vi "Stem Page.vi"() -> ()   [LabVIEW 2020, in "3D Stem.lvclass"]
uses:
  <vilib>/Math Plots/3D Math Plots/3D Stem/3D Stem/3D Stem.lvclass
  <vilib>/Math Plots/3D Math Plots/3D Stem/3D Stem/Typedef/3D Stem Property Array.ctl
  <vilib>/Math Plots/3D Math Plots/3D Stem/3D Stem/Typedef/3D Stem Property.ctl
  <vilib>/Math Plots/3D Math Plots/3D Plot/3D Plot/Typedef/Sprite Type.ctl
  <vilib>/Math Plots/3D Math Plots/3D Plot/3D Plot/Typedef/Color Ramp Cluster.ctl
  <vilib>/Math Plots/3D Math Plots/3D Plot/3D Plot/Typedef/Line Type.ctl
  <vilib>/Math Plots/3D Math Plots/3D Plot/3D Plot/Typedef/Dialog State.ctl
  <vilib>/Math Plots/3D Math Plots/3D Plot/3D Plot/Typedef/Temp Scene State.ctl
  <vilib>/Math Plots/3D Math Plots/3D Plot/3D Plot/Typedef/Temp Scene Property Action.ctl
  <vilib>/Math Plots/3D Math Plots/3D Plot/3D Plot/3D Plot.lvclass
panel:
  in  "Point Size":sgl caption="Point size" min=0.001 step=1
  in  "Point Style":u16(ring) caption="Point style"
  in  "Line Width":sgl=0.001 caption="Line width" min=0.001 step=1
  in  "Antialiasing":bool
  in  "Line Style":u16(ring) caption="Line style"
  in  "Line Color":u32(colorbox) caption="Line color"
  out "Stem Property Out":T1
  in  "Stem Property In":T1
  out "Color Ramp":dbl[][](graph)
  in  "Color Map Style":u16(ring) caption="Color map style" items=["None ", "Shaded", "Color spectrum", "Grey scale", "Custom"]
  in  "YZ Plane Projection":bool caption="YZ plane projection"
  in  "XZ Plane Projection":bool caption="XZ plane projection"
  in  "XY Plane Projection":bool caption="XY  plane projection"
  in  "Coordinate System":u16(ring) caption="Coordinate system" items=["Cartesian", "Cylindrical", "Spherical"]
  in  "Plot Opacity":sgl(slide) caption="Plot opacity(%)" min=0 max=100 scale=0.0..100.0
  in  "Plot List":i32(listbox)
  in  "Ramp Edit":bool caption="Ramp edit"
  in  "Move Down":bool
  in  "Move Up":bool
  in  "Delete":bool
  in  "New":bool
  in  "Event Registration":refnum<event-registration>
  # "Stem"
  # "General"
  # "Projection"
  # "Color Ramp"
  # "Stem Line"
  # "Stem Point"
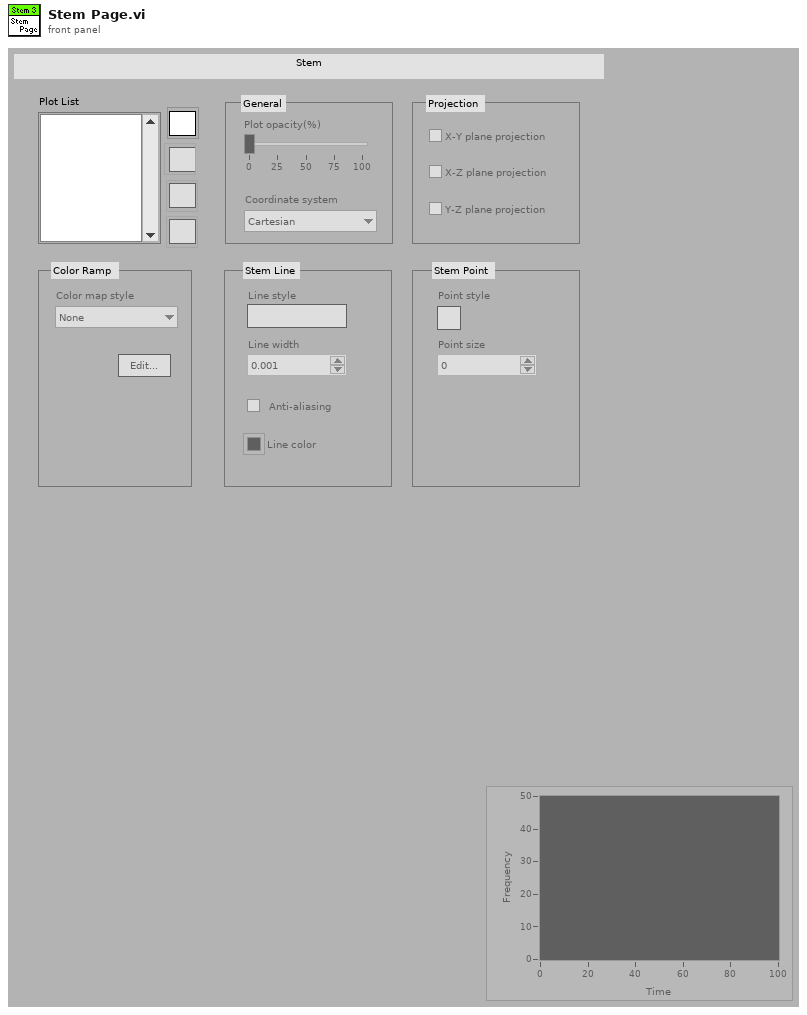
[diagram p1: front panel]
types:
  T1 = typedef "3D Stem.lvclass/3D Stem Property Array.ctl" = T2[]
  T2 = typedef "3D Stem.lvclass/3D Stem Property.ctl" = cluster{"General Property":cluster{"Plot Name":string, "Coordinate System":enum16{"Cartesian", "Cylindrical", "Spherical"}, "Opacity":sgl}, "Projection Property":cluster{"Draw XY":bool, "Draw YZ":bool, "Draw XZ":bool}, "Plot Property":cluster{"Sprite Type":T3, "Point Size":sgl, "Color Ramp Cluster":T4, "Line Style":T5, "Line Width":sgl, "Line Color":u32, "Antialiasing":bool}}
  T3 = typedef "3D Plot.lvclass/Sprite Type.ctl" = enum16{"None", "Empty Square", "Solid Square", "Empty Diamond", "Solid Diamond", "Empty Circle", "Solid Circle", "Asterisk", "Bold X", "Wireframe Sphere", "Solid Sphere", "Wireframe Cube", "Solid Cube"}
  T4 = typedef "3D Plot.lvclass/Color Ramp Cluster.ctl" = cluster{"Color Ramp Style":enum16{"None", "Shaded", "Color spectrum", "Grey scale", "Custom"}, "Color Ramp Array":u32[], "Color Ramp Index":i32[], "Interpolate?":bool, "Logarithm?":bool}
  T5 = typedef "3D Plot.lvclass/Line Type.ctl" = enum16{"None", "Solid", "Dash", "Dot", "Dash Dot"}
  T6 = typedef "3D Plot.lvclass/Dialog State.ctl" = enum16{"Initialize", "Read Porperty", "Write Property", "Idle", "Exit"}
  T7 = typedef "3D Plot.lvclass/Temp Scene State.ctl" = enum16{"Create", "Update Scene", "Get Plot Representation", "Destory"}
  T8 = typedef "3D Plot.lvclass/Temp Scene Property Action.ctl" = enum16{"Graph Property", "Light Property", "Axis Property", "Value Pair Property", "Format Property", "Cursor Property", "Plot Specific Property"}
  T9 = typedef "3D Plot.lvclass/Multiplot Representation.ctl" = cluster{"Plot Represention Array":T10[], "Max Range":T11}
  T10 = typedef "3D Plot.lvclass/Plot Representation.ctl" = cluster{"Plot ID":i32, "Plot Range":T11, "Mesh Data":T12, "Dimension":cluster{"X Dimension":i32, "Y Dimension":i32}, "Ramp Range":T11}
  T11 = typedef "3D Plot.lvclass/Range Clusters.ctl" = cluster{"X Range":cluster{"Max X":sgl, "Min X":sgl}, "Y Range":cluster{"Max Y":sgl, "Min Y":sgl}, "Z Range":cluster{"Max Z":sgl, "Min Z":sgl}}
  T12 = typedef "3D Plot.lvclass/Mesh Data.ctl" = cluster{"Index Array":u32[], "Vertex Array":cluster{"X":sgl, "Y":sgl, "Z":sgl}[], "Normal Array":cluster{"X":sgl, "Y":sgl, "Z":sgl}[], "Color Index Array":i32[]}
  T13 = enum16{"None", "Shaded", "Color spectrum", "Grey scale", "Custom"}
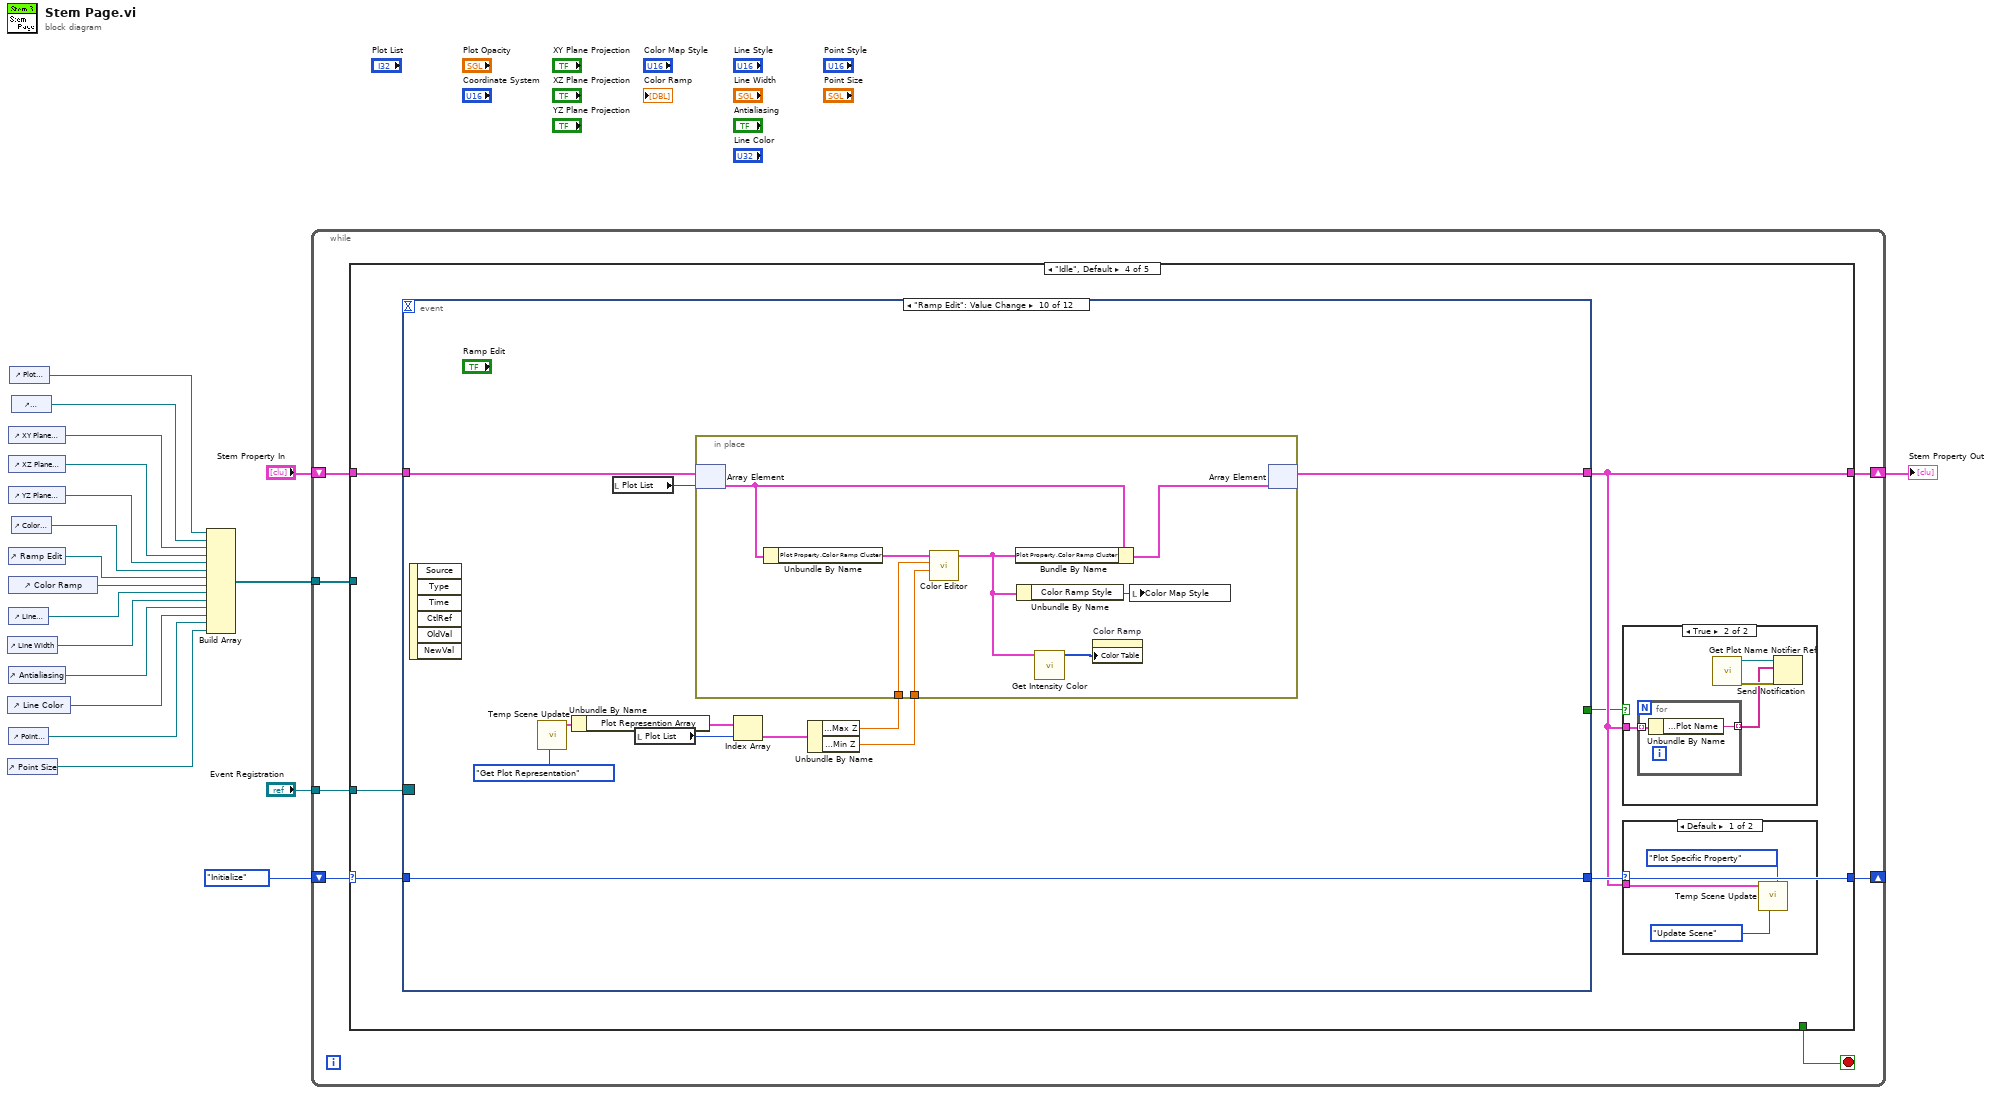
[diagram p0: block diagram]
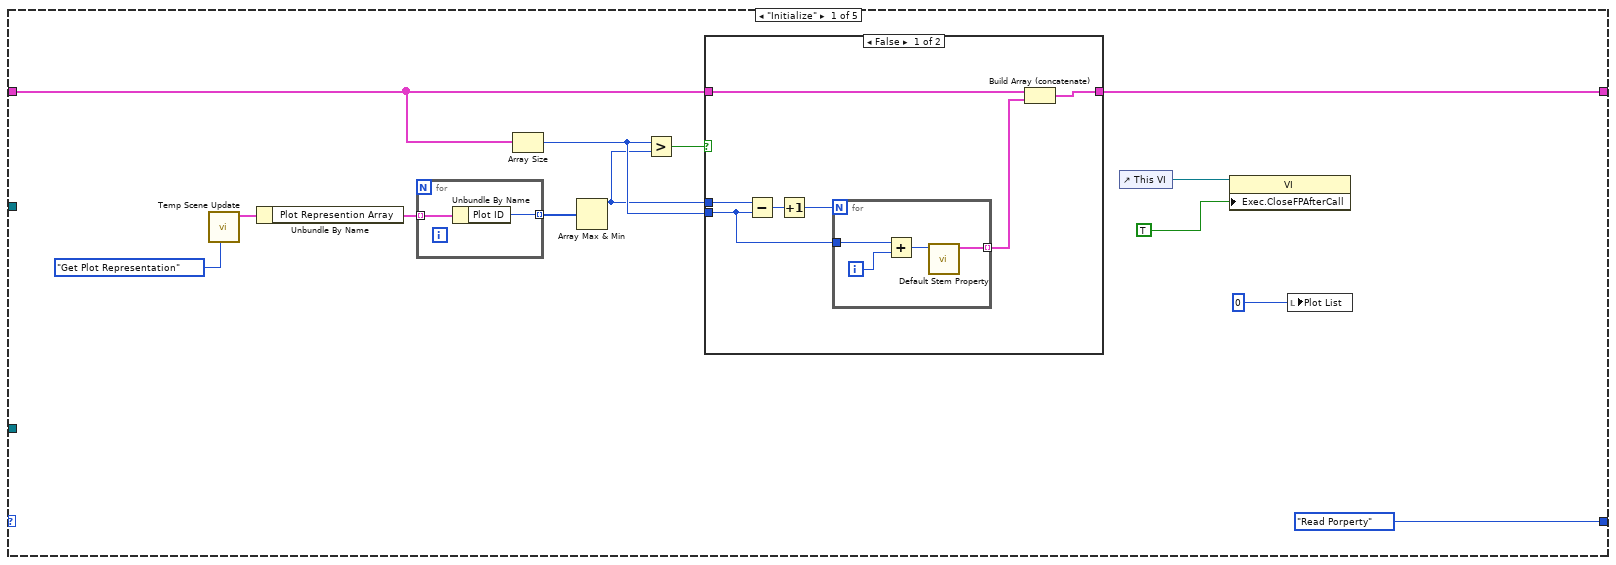
[diagram p2: hidden frame]
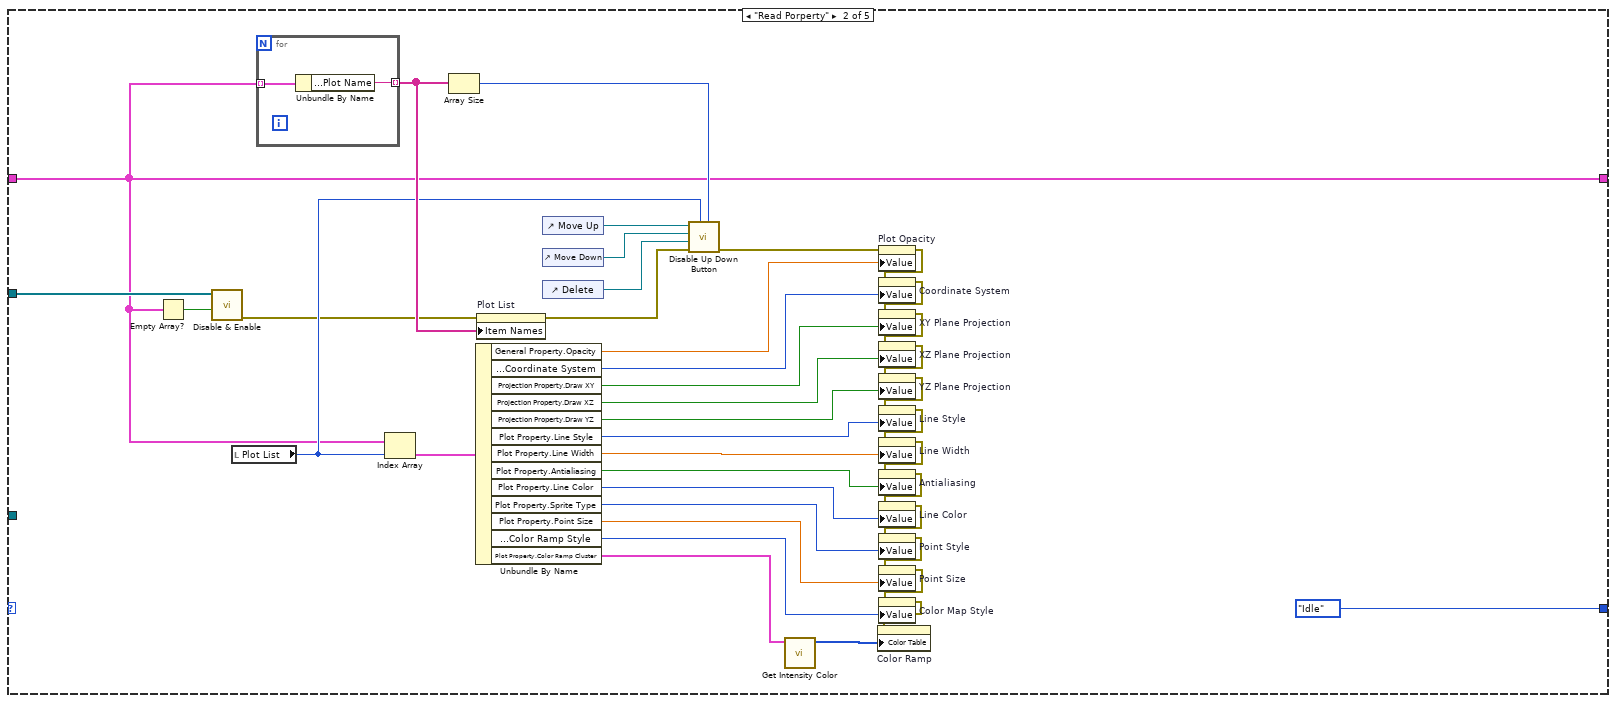
[diagram p4: hidden frame]
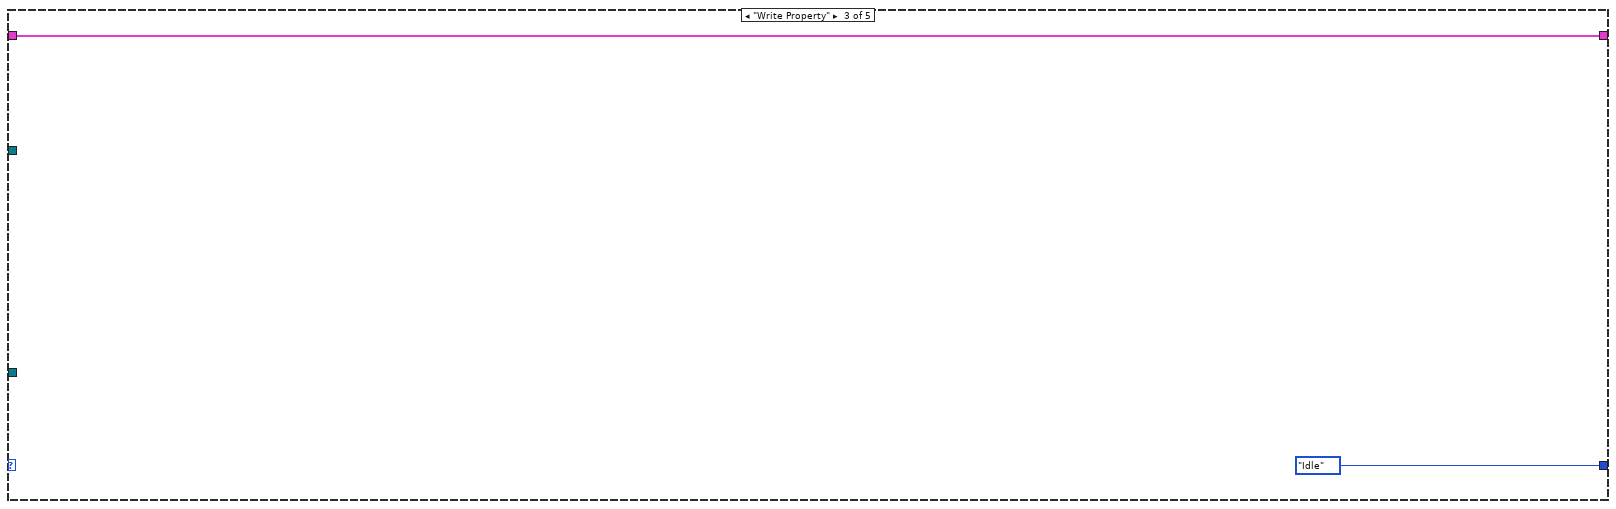
[diagram p5: hidden frame]
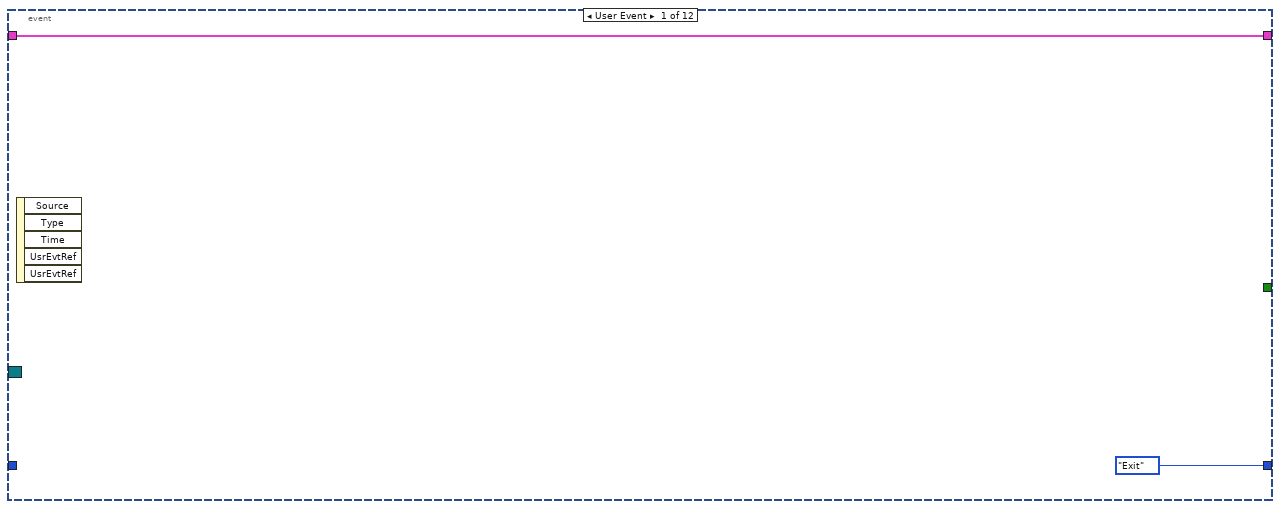
[diagram p8: hidden frame]
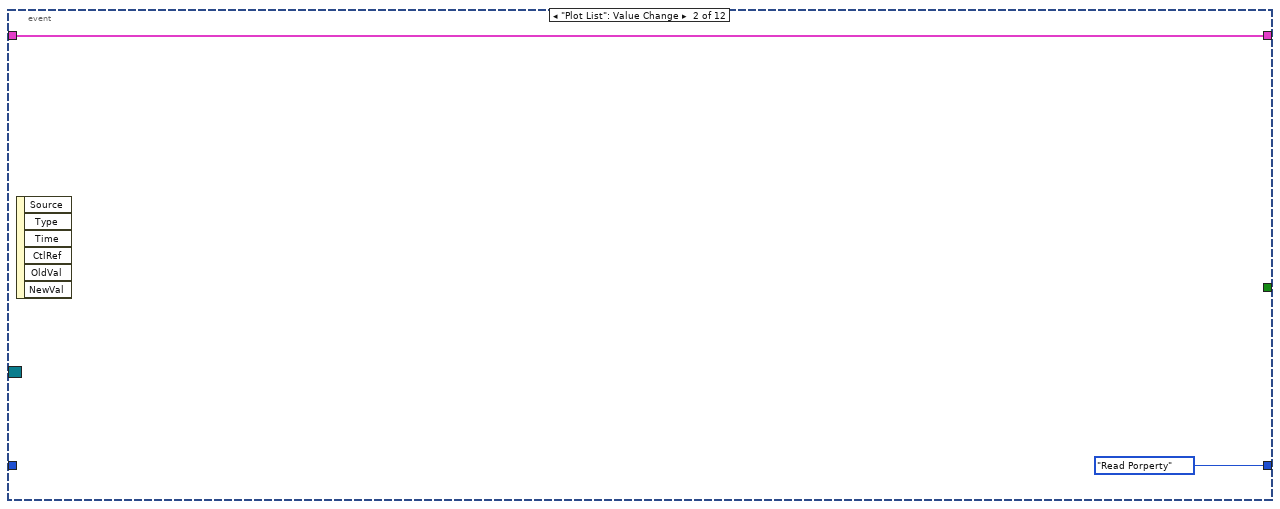
[diagram p9: hidden frame]
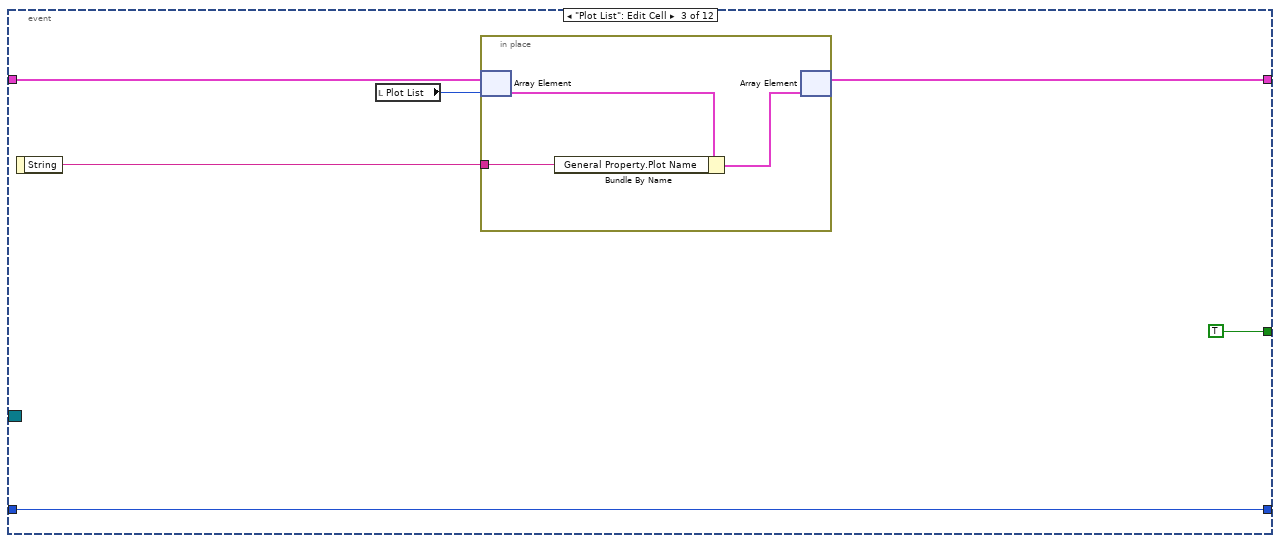
[diagram p10: hidden frame]
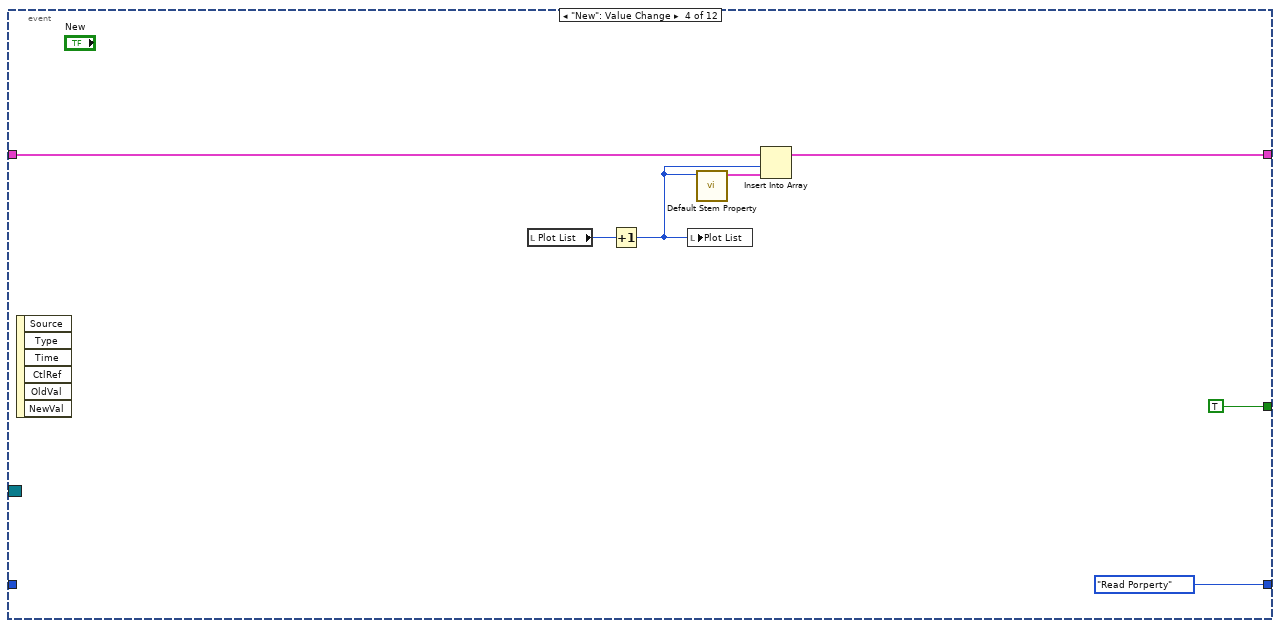
[diagram p11: hidden frame]
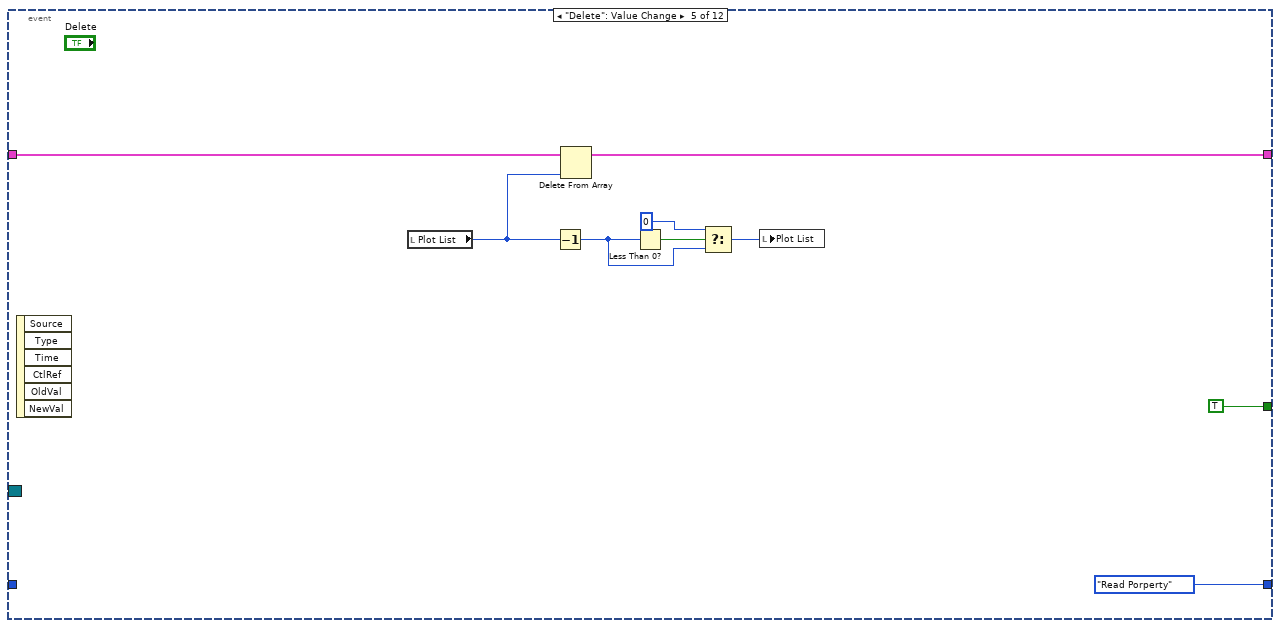
[diagram p12: hidden frame]
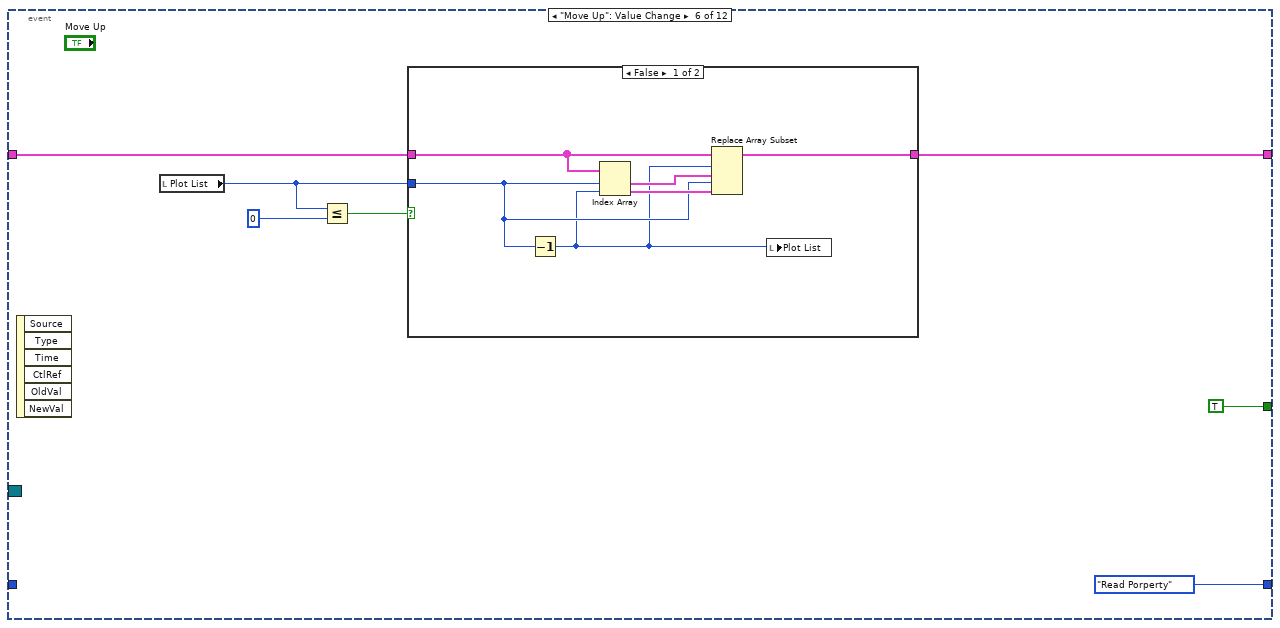
[diagram p13: hidden frame]
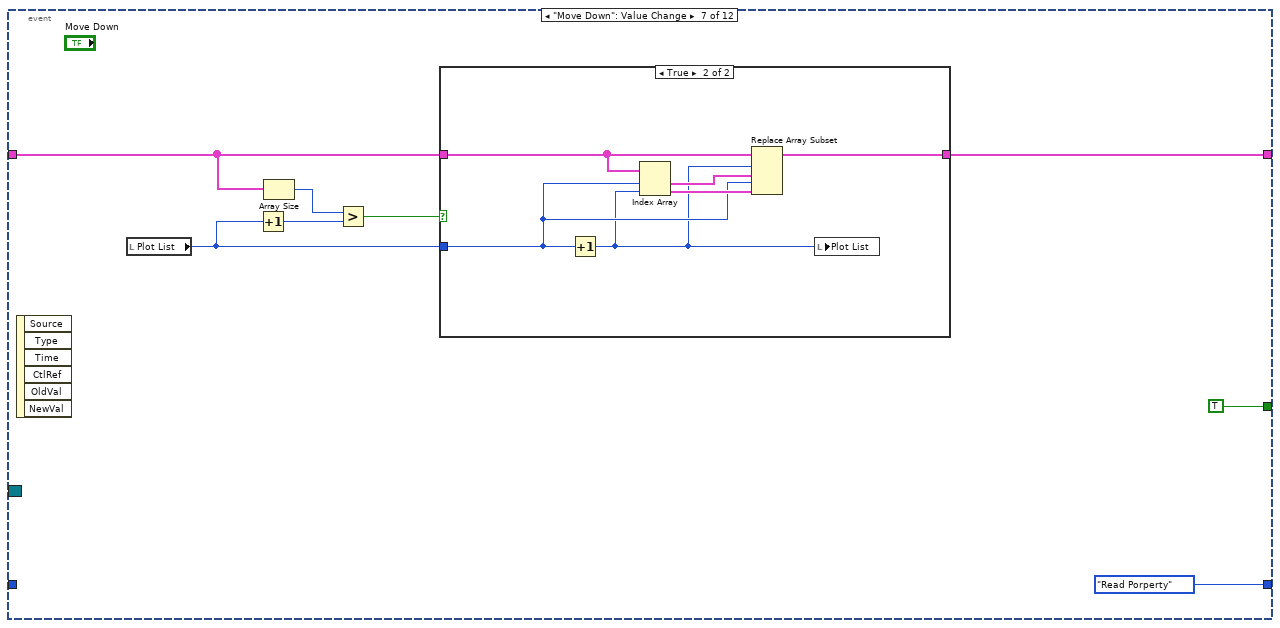
[diagram p15: hidden frame]
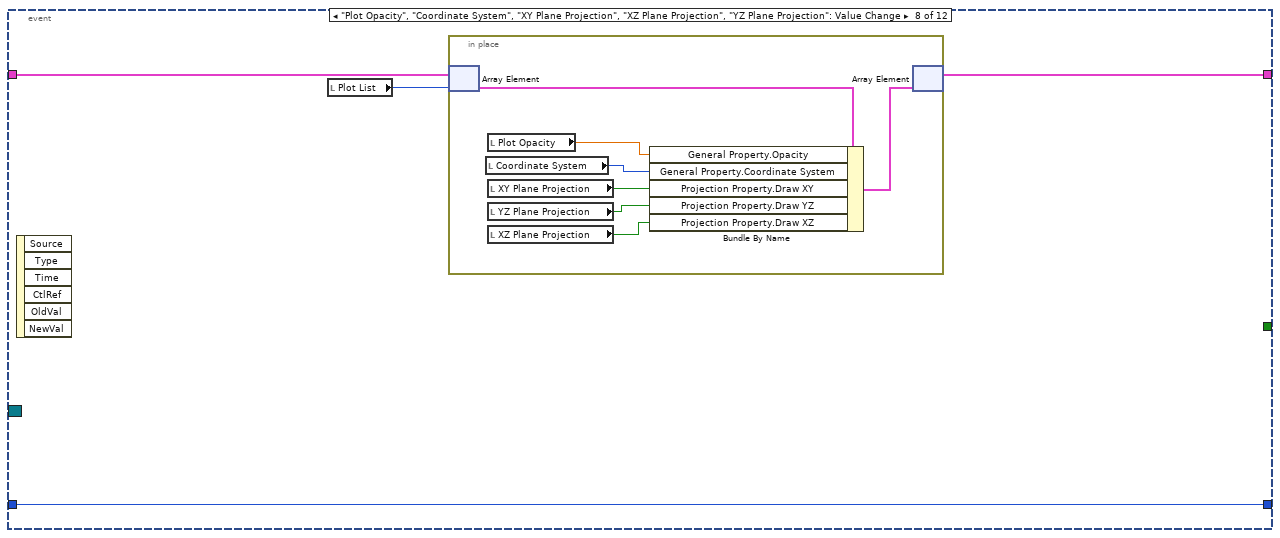
[diagram p17: hidden frame]
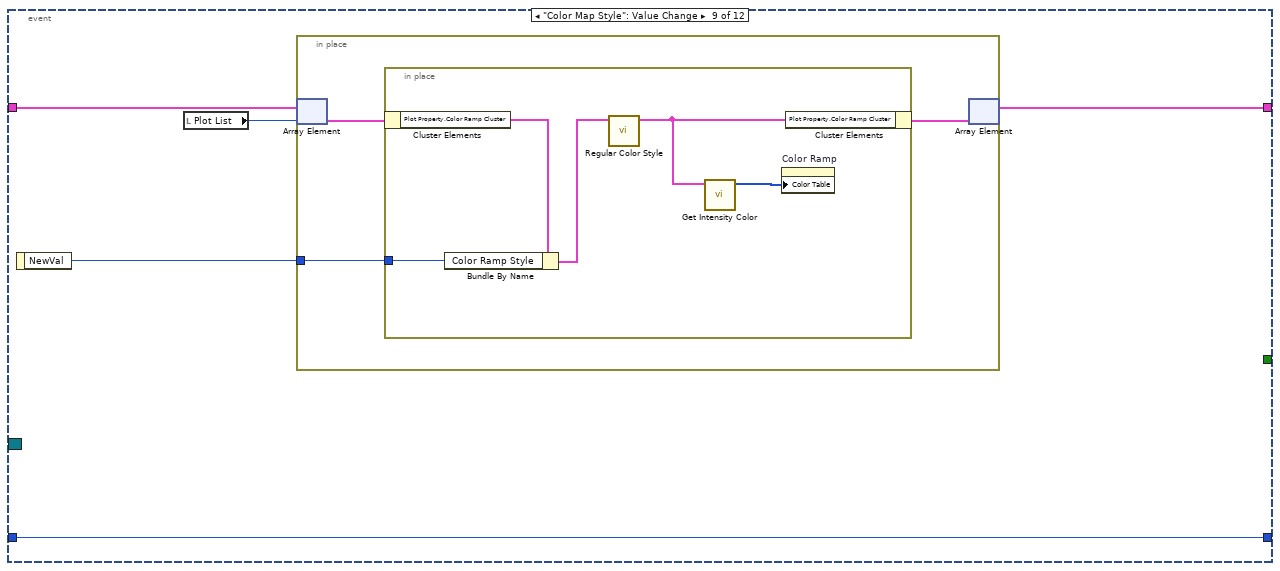
[diagram p18: hidden frame]
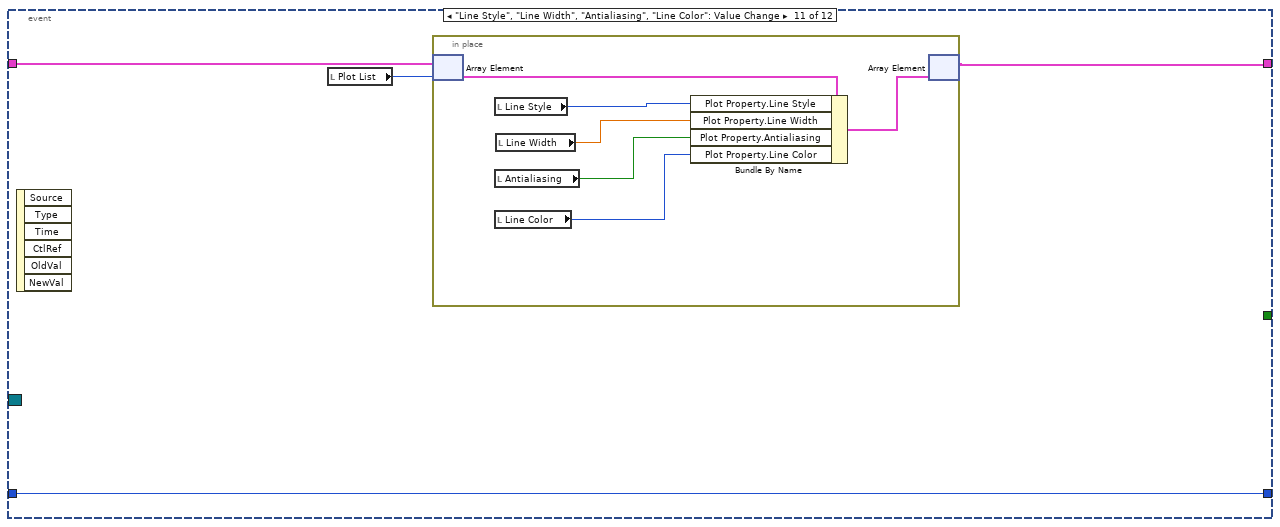
[diagram p19: hidden frame]
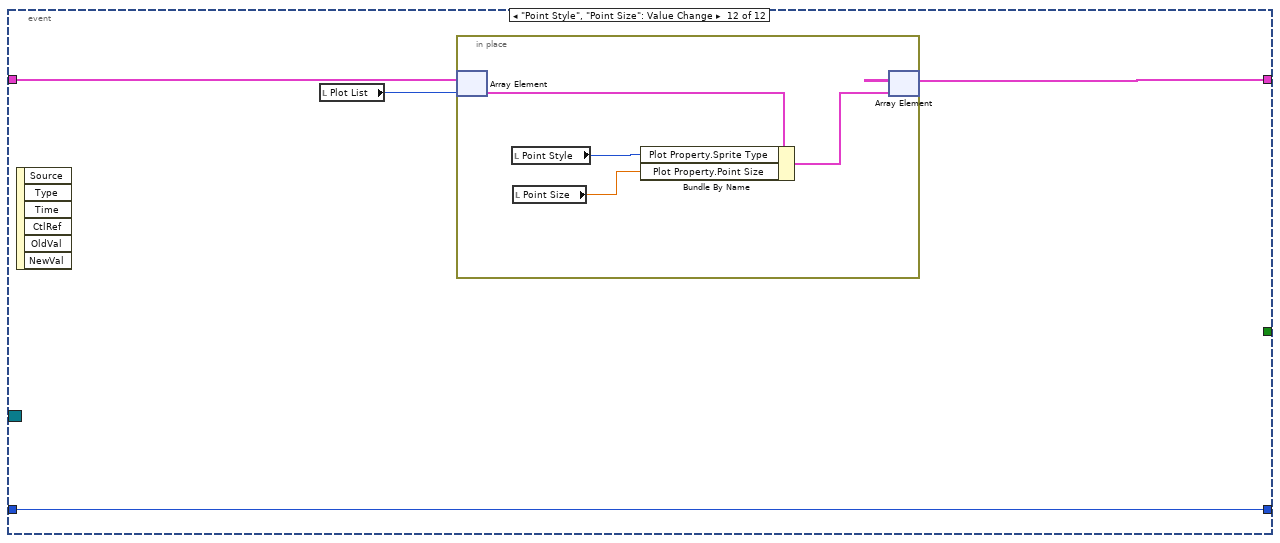
[diagram p20: hidden frame]
diagram:
  n1 = control-ref of="Line Width"() -> (w6:refnum<vi>)
  n2 = control-ref of="Line Color"() -> (w4:refnum<vi>)
  n3 = control-ref of="Point Size"() -> (w2:refnum<vi>)
  n4 = control-ref of="XY Plane Projection"() -> (w13:refnum<vi>)
  n5 = control-ref of="XZ Plane Projection"() -> (w12:refnum<vi>)
  n6 = control-ref of="YZ Plane Projection"() -> (w11:refnum<vi>)
  n7 = control-ref of="Ramp Edit"() -> (w9:refnum<vi>)
  n8 = control-ref of="Color Ramp"() -> (w8:refnum<vi>)
  n9 = control-ref of="Line Style"() -> (w7:refnum<vi>)
  n10 = control-ref of="Antialiasing"() -> (w5:refnum<vi>)
  n11 = control-ref of="Point Style"() -> (w3:refnum<vi>)
  n12 = control-ref of="Plot Opacity"() -> (w15:refnum<vi>)
  n13 = control-ref of="Coordinate System"() -> (w14:refnum<vi>)
  n14 = control-ref of="Color Map Style"() -> (w10:refnum<vi>)
  n15 = Build Array(w15, w14, w13, w12, w11, w10, w9, w8, w7, w6, w5, w4, w3, w2) -> (w1:refnum<vi>[])
  n16 = while {
    shift-right: [w25] -> w16
    shift-left: "Stem Property In" -> [w26]
    shift-right: [w21] -> _
    shift-left: Dialog_State."Initialize" -> [w24]
    tunnel: "Event Registration" -> [w22]
    tunnel: w1 -> [w20]
    stop <- w23 stop-if-true
    n17 = case shown="\"Idle\", Default" w24 {
      selector: w24 -> [_ _ _ w101 _]
      tunnel: w26 -> [w29 w80 w96 w103 w232]
      tunnel: [w28 w80 w96 w99 w232] -> w25
      tunnel: [Dialog_State."Read Porperty" Dialog_State."Idle" Dialog_State."Idle" w100 Dialog_State."Exit"] -> w21
      tunnel: [_ _ _ _ TRUE] -> w23
      tunnel: w22 -> [_ _ _ w102 _]
      tunnel: w20 -> [_ w81 _ _ _]
      frame "Initialize" {
        n18 = call <vilib>:"Temp Scene Update.vi"("State"=Temp_Scene_State."Get Plot Representation") -> ("Multiplot Representation"=w34:T9)  [unwired: 5 in, 5 out]
        n19 = Unbundle By Name(w34) -> ("Plot Represention Array"=w27:T10[])
        n20 = for {
          tunnel: w27 -> [w53] mode=indexing
          tunnel: [w52] -> w33 mode=indexing
          n21 = Unbundle By Name(w53) -> ("Plot ID"=w52:i32)
        }
        n22 = Array Size(array=w29) -> (size(s)=w31:i32)
        n23 = Array Max & Min(array=w33) -> (max value=w30:i32)  [unwired: 3 out]
        n24 = Greater?(x=w31, y=w30) -> (0:w32:bool)
        n25 = case shown="False" w32 {
          tunnel: [w44 w51] -> w28
          tunnel: w29 -> [w46 w51]
          tunnel: w31 -> [w40 _]
          tunnel: w30 -> [w41 _]
          frame False {
            n26 = Subtract(x=w41, y=w40) -> (x-y=w43:i32)
            n27 = Increment(x=w43) -> (x+1=w42:i32)
            n28 = for {
              N: w42 -> [_]
              tunnel: w40 -> [w49]
              tunnel: [w47] -> w45 mode=indexing
              i -> [w50]
              n29 = Add(x=w49, y=w50) -> (x+y=w48:i32)
              n30 = call <vilib>:"Default Stem Property.vi"("Plot ID"=w48) -> ("Default Property"=w47:T2)  [unwired: 10 out]
            }
            n31 = Build Array (concatenate)(w46, w45) -> (w44:T1)
          }
          frame True {
          }
        }
        n32 = control-ref of="This VI"() -> (w38:refnum<vi>)
        n33 = property class="VI"(reference=w38, "Exec.CloseFPAfterCall"=TRUE ("Execution:Close After Call")) -> ()  [unwired: 1 in, 2 out]
        n34 = local write "Plot List"(0 ("Plot List")) -> ()
      }
      frame "Read Porperty" {
        n35 = Empty Array?(array=w80) -> (empty?=w82:bool)
        n36 = call <vilib>:"Disable & Enable.vi"("Disabled?"=w82, "Control Ref Array"=w81) -> ("error out"=w79:errorcluster)  [unwired: 1 in, 8 out]
        n37 = local read "Plot List"() -> (w83:i32)
        n38 = for {
          tunnel: w80 -> [w95] mode=indexing
          tunnel: [w94] -> w85 mode=indexing
          n39 = Unbundle By Name(w95) -> ("General Property.Plot Name"=w94:string)
        }
        n40 = Index Array(array=w80, index=w83) -> (element=w92:T2)
        n41 = Array Size(array=w85) -> (size(s)=w86:i32)
        n42 = Unbundle By Name(w92) -> ("General Property.Opacity"=w70:sgl, "General Property.Coordinate System"=w69:enum16{"Cartesian", "Cylindrical", "Spherical"}, "Projection Property.Draw XY"=w68:bool, "Projection Property.Draw XZ"=w67:bool, "Projection Property.Draw YZ"=w66:bool, "Plot Property.Line Style"=w65:T5, "Plot Property.Line Width"=w64:sgl, "Plot Property.Antialiasing"=w63:bool, "Plot Property.Line Color"=w61:u32, "Plot Property.Sprite Type"=w60:T3, "Plot Property.Point Size"=w59:sgl, "Plot Property.Color Ramp Cluster.Color Ramp Style"=w58:T13, "Plot Property.Color Ramp Cluster"=w91:T4)
        n43 = property on="Plot List" class="LstBox (strict)"(error in=w79, "Item Names"=w85) -> (error out=w84:errorcluster)  [unwired: 1 in, 1 out]
        n44 = control-ref of="Move Up"() -> (w87:refnum<vi>)
        n45 = control-ref of="Move Down"() -> (w88:refnum<vi>)
        n46 = control-ref of="Delete"() -> (w89:refnum<vi>)
        n47 = call <vilib>:"Disable Up Down Button.vi"("Length"=w86, "Index"=w83, "error in (no error)"=w84, "Delete Ref"=w89, "Move Down Ref"=w88, "Move Up Ref"=w87) -> ("error out"=w55:errorcluster)  [unwired: 5 out]
        n48 = call <vilib>:"Get Intensity Color.vi"("Color Ramp Cluster"=w91) -> ("Intensity Color"=w90:u32[])  [unwired: 4 in, 6 out]
        n49 = property on="Plot Opacity" class="Slide (strict)"(error in=w55, "Value"=w70) -> (error out=w78:errorcluster)  [unwired: 1 in, 1 out]
        n50 = property on="Coordinate System" class="Ring (strict)"(error in=w78, "Value"=w69) -> (error out=w77:errorcluster)  [unwired: 1 in, 1 out]
        n51 = property on="XY Plane Projection" class="Bool (strict)"(error in=w77, "Value"=w68) -> (error out=w76:errorcluster)  [unwired: 1 in, 1 out]
        n52 = property on="XZ Plane Projection" class="Bool (strict)"(error in=w76, "Value"=w67) -> (error out=w75:errorcluster)  [unwired: 1 in, 1 out]
        n53 = property on="YZ Plane Projection" class="Bool (strict)"(error in=w75, "Value"=w66) -> (error out=w74:errorcluster)  [unwired: 1 in, 1 out]
        n54 = property on="Line Style" class="Ring (strict)"(error in=w74, "Value"=w65) -> (error out=w73:errorcluster)  [unwired: 1 in, 1 out]
        n55 = property on="Line Width" class="DigNum (strict)"(error in=w73, "Value"=w64) -> (error out=w72:errorcluster)  [unwired: 1 in, 1 out]
        n56 = property on="Antialiasing" class="Bool (strict)"(error in=w72, "Value"=w63) -> (error out=w57:errorcluster)  [unwired: 1 in, 1 out]
        n57 = property on="Line Color" class="ColBox"(error in=w57, "Value"=w61) -> (error out=w56:errorcluster)  [unwired: 1 in, 1 out]
        n58 = property on="Point Style" class="Ring (strict)"(error in=w56, "Value"=w60) -> (error out=w62:errorcluster)  [unwired: 1 in, 1 out]
        n59 = property on="Point Size" class="DigNum (strict)"(error in=w62, "Value"=w59) -> (error out=w71:errorcluster)  [unwired: 1 in, 1 out]
        n60 = property on="Color Map Style" class="Ring (strict)"(error in=w71, "Value"=w58) -> (error out=w54:errorcluster)  [unwired: 1 in, 1 out]
        n61 = property on="Color Ramp" class="IntGraph (strict)"(error in=w54, "Color Table"=w90) -> ()  [unwired: 1 in, 2 out]
      }
      frame "Write Property" {
      }
      frame "Idle", Default {
        n62 = event shown="[9] \"Ramp Edit\": Value Change" {
          selector: w102 -> [_ _ _ _ _ _ _ _ _ _ _ _]
          dyn-events: _ -> [_ _ _ _ _ _ _ _ _ _ _ _]
          timeout: _ -> [_ _ _ _ _ _ _ _ _ _ _ _]
          tunnel: w103 -> [w114 w116 w120 w130 w139 w143 w158 w172 w185 w203 w215 w225]
          tunnel: [w114 w116 w119 w129 w140 w144 w157 w171 w182 w202 w214 w224] -> w99
          tunnel: [Dialog_State."Exit" Dialog_State."Read Porperty" w118 Dialog_State."Read Porperty" Dialog_State."Read Porperty" Dialog_State."Read Porperty" Dialog_State."Read Porperty" w174 w186 w205 w217 w226] -> w100
          tunnel: w101 -> [_ _ w118 _ _ _ _ w174 w186 w205 w217 w226]
          tunnel: [_ _ TRUE TRUE TRUE TRUE TRUE _ _ _ _ _] -> w98
          event User Event {
            n63 = event-data() -> ()  [unwired: 6 out]
          }
          event "Plot List": Value Change {
            n64 = event-data() -> ()  [unwired: 7 out]
          }
          event "Plot List": Edit Cell {
            n65 = event-data() -> ("String"=w121:string)  [unwired: 1 out]
            n66 = local read "Plot List"() -> (w122:i32)
            n67 = in-place {
              in-place-border: w121 -> [w123]
              n68 = in-place-array #1(w120, w122) -> (w125:T2)
              n69 = Bundle By Name(cluster=w125, "General Property.Plot Name"=w123) -> (w124:T2)
              n70 = in-place-array #1(w124) -> (w119:T1)  [unwired: 1 out]
            }
          }
          event "New": Value Change {
            n71 = event-data() -> ()  [unwired: 7 out]
            n72 = local read "Plot List"() -> (w131:i32)
            n73 = Increment(x=w131) -> (x+1=w127:i32)
            n74 = local write "Plot List"(w127) -> ()
            n75 = call <vilib>:"Default Stem Property.vi"("Plot ID"=w127) -> ("Default Property"=w126:T2)  [unwired: 10 out]
            n76 = Insert Into Array(array=w130, index=w127, new element=w126) -> (w129:T1)
          }
          event "Delete": Value Change {
            n77 = event-data() -> ()  [unwired: 7 out]
            n78 = local read "Plot List"() -> (w135:i32)
            n79 = Decrement(x=w135) -> (x-1=w136:i32)
            n80 = Delete From Array(array=w139, index=w135) -> (array with subset deleted=w140:T1)  [unwired: 1 in, 1 out]
            n81 = Less Than 0?(x=w136) -> (x < 0?=w138:bool)
            n82 = Select(t=0, s=w138, f=w136) -> (s? t:f=w134:i32)
            n83 = local write "Plot List"(w134) -> ()
          }
          event "Move Up": Value Change {
            n84 = event-data() -> ()  [unwired: 7 out]
            n85 = local read "Plot List"() -> (w145:i32)
            n86 = Less Or Equal?(x=w145, y=0) -> (x <= y?=w146:bool)
            n87 = case shown="False" w146 {
              tunnel: w143 -> [w152 w155]
              tunnel: [w151 w155] -> w144
              tunnel: w145 -> [w150 _]
              frame False {
                n88 = Decrement(x=w150) -> (x-1=w149:i32)
                n89 = Index Array(array=w152, index #1=w150, index #2=w149) -> (element #1=w154:T2, element #2=w153:T2)
                n90 = Replace Array Subset(array=w152, new element #1=w154, index #1=w149, new element #2=w153, index #2=w150) -> (w151:T1)
                n91 = local write "Plot List"(w149) -> ()
              }
              frame True {
                # "List value is less or equal to 0.\nThe active item is in the top of the list."
              }
            }
          }
          event "Move Down": Value Change {
            n92 = event-data() -> ()  [unwired: 7 out]
            n93 = local read "Plot List"() -> (w159:i32)
            n94 = Increment(x=w159) -> (x+1=w161:i32)
            n95 = Array Size(array=w158) -> (size(s)=w162:i32)
            n96 = Greater?(x=w162, y=w161) -> (0:w160:bool)
            n97 = case shown="True" w160 {
              tunnel: w158 -> [w164 w168]
              tunnel: [w164 w167] -> w157
              tunnel: w159 -> [_ w166]
              frame False {
                # "List value +1 is not less array length.\nThe active item is in the buttom of the list."
              }
              frame True {
                n98 = Increment(x=w166) -> (x+1=w165:i32)
                n99 = Index Array(array=w168, index #1=w166, index #2=w165) -> (element #1=w170:T2, element #2=w169:T2)
                n100 = Replace Array Subset(array=w168, new element #1=w170, index #1=w165, new element #2=w169, index #2=w166) -> (w167:T1)
                n101 = local write "Plot List"(w165) -> ()
              }
            }
          }
          event "Plot Opacity", "Coordinate System", "XY Plane Projection", "XZ Plane Projection", "YZ Plane Projection": Value Change {
            n102 = event-data() -> ()  [unwired: 7 out]
            n103 = local read "Plot List"() -> (w173:i32)
            n104 = in-place {
              n105 = in-place-array #2(w172, w173) -> (w177:T2)
              n106 = local read "Coordinate System"() -> (w175:u16)
              n107 = local read "Plot Opacity"() -> (w181:sgl)
              n108 = local read "XY Plane Projection"() -> (w180:bool)
              n109 = local read "YZ Plane Projection"() -> (w178:bool)
              n110 = local read "XZ Plane Projection"() -> (w179:bool)
              n111 = Bundle By Name(cluster=w177, "General Property.Opacity"=w181, "General Property.Coordinate System"=w175, "Projection Property.Draw XY"=w180, "Projection Property.Draw YZ"=w178, "Projection Property.Draw XZ"=w179) -> (w176:T2)
              n112 = in-place-array #2(w176) -> (w171:T1)  [unwired: 1 out]
            }
          }
          event "Color Map Style": Value Change {
            n113 = event-data() -> ("NewVal"=w183:u16)  [unwired: 1 out]
            n114 = local read "Plot List"() -> (w184:i32)
            n115 = in-place {
              in-place-border: w183 -> [w188]
              n116 = in-place-array #3(w185, w184) -> (w189:T2)
              n117 = in-place {
                in-place-border: w188 -> [w193]
                n118 = in-place-cluster #4(w189) -> ("Plot Property.Color Ramp Cluster"=w194:T4)
                n119 = Bundle By Name(cluster=w194, "Color Ramp Style"=w193) -> (w192:T4)
                n120 = call <vilib>:"Regular Color Style.vi"("Color Ramp Cluster in"=w192) -> ("Color Ramp Cluster out"=w190:T4)  [unwired: 10 in]
                n121 = call <vilib>:"Get Intensity Color.vi"("Color Ramp Cluster"=w190) -> ("Intensity Color"=w191:u32[])  [unwired: 4 in, 6 out]
                n122 = property on="Color Ramp" class="IntGraph (strict)"("Color Table"=w191) -> ()  [unwired: 2 in, 2 out]
                n123 = in-place-cluster #4("Plot Property.Color Ramp Cluster"=w190) -> (w187:T2)
              }
              n124 = in-place-array #3(w187) -> (w182:T1)  [unwired: 1 out]
            }
          }
          event "Ramp Edit": Value Change {
            n125 = event-data() -> ()  [unwired: 7 out]
            n126 = call <vilib>:"Temp Scene Update.vi"("State"=Temp_Scene_State."Get Plot Representation") -> ("Multiplot Representation"=w198:T9)  [unwired: 5 in, 5 out]
            n127 = Unbundle By Name(w198) -> ("Plot Represention Array"=w195:T10[])
            n128 = local read "Plot List"() -> (w204:i32)
            n129 = local read "Plot List"() -> (w201:i32)
            n130 = Index Array(array=w195, index=w201) -> (element=w200:T10)
            n131 = Unbundle By Name(w200) -> ("Plot Range.Z Range.Max Z"=w197:sgl, "Plot Range.Z Range.Min Z"=w196:sgl)
            n132 = in-place {
              in-place-border: w197 -> [w209]
              in-place-border: w196 -> [w208]
              n133 = in-place-array #5(w203, w204) -> (w212:T2)
              n134 = Unbundle By Name(w212) -> ("Plot Property.Color Ramp Cluster"=w211:T4)
              n135 = call <vilib>:"Color Editor.vi"("Min"=w208, "Max"=w209, "Color Ramp Cluster in"=w211) -> ("Color Ramp Cluster out"=w207:T4)  [unwired: 3 in, 5 out]
              n136 = Bundle By Name(cluster=w212, "Plot Property.Color Ramp Cluster"=w207) -> (w213:T2)
              n137 = Unbundle By Name(w207) -> ("Color Ramp Style"=w206:T13)
              n138 = call <vilib>:"Get Intensity Color.vi"("Color Ramp Cluster"=w207) -> ("Intensity Color"=w210:u32[])  [unwired: 4 in, 6 out]
              n139 = property on="Color Ramp" class="IntGraph (strict)"("Color Table"=w210) -> ()  [unwired: 2 in, 2 out]
              n140 = local write "Color Map Style"(w206) -> ()
              n141 = in-place-array #5(w213) -> (w202:T1)  [unwired: 1 out]
            }
          }
          event "Line Style", "Line Width", "Antialiasing", "Line Color": Value Change {
            n142 = event-data() -> ()  [unwired: 7 out]
            n143 = local read "Plot List"() -> (w216:i32)
            n144 = in-place {
              n145 = in-place-array #6(w215, w216) -> (w220:T2)
              n146 = local read "Line Style"() -> (w223:u16)
              n147 = local read "Antialiasing"() -> (w221:bool)
              n148 = local read "Line Color"() -> (w218:u32)
              n149 = local read "Line Width"() -> (w222:sgl)
              n150 = Bundle By Name(cluster=w220, "Plot Property.Line Style"=w223, "Plot Property.Line Width"=w222, "Plot Property.Antialiasing"=w221, "Plot Property.Line Color"=w218) -> (w219:T2)
              n151 = in-place-array #6(w219) -> (w214:T1)  [unwired: 1 out]
            }
          }
          event "Point Style", "Point Size": Value Change {
            n152 = event-data() -> ()  [unwired: 7 out]
            n153 = local read "Plot List"() -> (w227:i32)
            n154 = in-place {
              n155 = in-place-array #7(w225, w227) -> (w231:T2)
              n156 = local read "Point Style"() -> (w228:u16)
              n157 = local read "Point Size"() -> (w229:sgl)
              n158 = Bundle By Name(cluster=w231, "Plot Property.Sprite Type"=w228, "Plot Property.Point Size"=w229) -> (w230:T2)
              n159 = in-place-array #7(w230) -> (w224:T1)  [unwired: 1 out]
            }
          }
        }
        n160 = case shown="True" w98 {
          tunnel: w99 -> [_ w104]
          frame False {
          }
          frame True {
            n161 = for {
              tunnel: w104 -> [w109] mode=indexing
              tunnel: [w108] -> w105 mode=indexing
              n162 = Unbundle By Name(w109) -> ("General Property.Plot Name"=w108:string)
            }
            n163 = call <vilib>:"Get Plot Name Notifier Ref.vi"() -> ("error out"=w107:errorcluster, "Plot Names Notifier Ref"=w106:refnum<notifier>)  [unwired: 1 in, 9 out]
            n164 = Send Notification(notification=w105, notifier=w106, error in (no error)=w107) -> ()  [unwired: 2 out]
          }
        }
        n165 = case shown="Default" w100 {
          tunnel: w99 -> [w112 _]
          frame Default {
            n166 = call <vilib>:"Temp Scene Update.vi"("Property Name"=Temp_Scene_Property_Action."Plot Specific Property", "State"=Temp_Scene_State."Update Scene", "Property In"=w112) -> ()  [unwired: 3 in, 6 out]
          }
          frame "Exit" {
          }
        }
      }
      frame "Exit" {
      }
    }
  }
  "Stem Property Out" <- w16
